vi "Raw To Scaled Value.vi"(1 "Scaling Constants":T1, 2 "u16 Raw Value":u16) -> (7 "dbl Scaled Value":dbl)   [LabVIEW 2021]
uses:
  <vilib>/myRIO/Common/Instrument Driver Framework/Utilities/typedefs/Analog Scaling Constants.ctl
panel:
  # "Converts raw ADC u16 value to scaled dbl value based on the scaling constants."
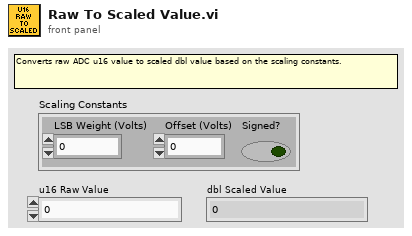
[diagram p1: front panel]
types:
  T1 = typedef "Analog Scaling Constants.ctl" = cluster{"LSB Weight (Volts)":dbl, "Offset (Volts)":dbl, "Signed?":bool}
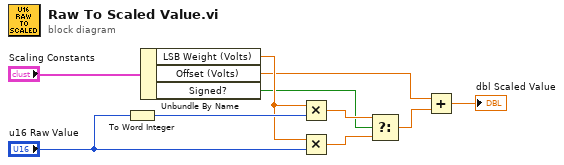
[diagram p0: block diagram]
diagram:
  n1 = To Word Integer(number="u16 Raw Value") -> (16bit integer=w8:i16)
  n2 = Unbundle By Name("Scaling Constants") -> ("LSB Weight (Volts)"=w7:dbl, "Offset (Volts)"=w4:dbl, "Signed?"=w1:bool)
  n3 = Multiply(x=w7, y=w8) -> (x*y=w6:dbl)
  n4 = Multiply(x=w7, y="u16 Raw Value") -> (x*y=w5:dbl)
  n5 = Select(t=w6, s=w1, f=w5) -> (s? t:f=w3:dbl)
  n6 = Add(x=w4, y=w3) -> (x+y=→"dbl Scaled Value":dbl)
